vi "Ballistics Message Center.vi"(0 "INI File Name":string="ballistic.ini") -> ()   [LabVIEW 2015]
uses:
  Instance           1 33Saved   Ballistics Message Center .vi
panel:
  in  "Save":bool
  out "Over 10":string="Not Due"
  out "Over 9":string="Not Due"
  out "Over 8":string="Not Due"
  out "Over 7":string="Not Due"
  out "Over 6":string="Not Due"
  out "Over 5":string="Not Due"
  out "Over 4":string="Not Due"
  out "Over 3":string="Not Due"
  out "Over 2":string="Not Due"
  out "Over 1":string="Not Due"
  in  "Date":string[](array[string])
  in  "Interval in Days":string[](array[string])
  in  "Message":string[](array[string])
  in  "No Alarms":bool
  in  "Edit File":bool
  out "RadioArray":cluster{bool, bool}[](array[cluster])=[{FALSE, TRUE}, {FALSE, TRUE}, {FALSE, TRUE}, {FALSE, TRUE}, {FALSE, TRUE}, {FALSE, TRUE}, {FALSE, TRUE}, {FALSE, TRUE}, {FALSE, TRUE}, {FALSE, TRUE}]
  in  "Remind 1":bool=TRUE
  in  "Completed 1":bool
  out "Date 10":string
  out "Date 9":string
  out "Date 8":string
  out "Date 7":string
  out "Date 6":string
  out "Date 5":string
  out "Date 4":string
  out "Date 3":string
  out "Date 2":string
  out "Date 1":string
  in  "Remind 10":bool=TRUE
  in  "Remind 9":bool=TRUE
  in  "Remind 8":bool=TRUE
  in  "Remind 7":bool=TRUE
  in  "Remind 6":bool=TRUE
  in  "Remind 5":bool=TRUE
  in  "Remind 4":bool=TRUE
  in  "Remind 3":bool=TRUE
  in  "Remind 2":bool=TRUE
  in  "Completed 10":bool
  in  "Completed 9":bool
  in  "Completed 8":bool
  in  "Completed 7":bool
  in  "Completed 6":bool
  in  "Completed 5":bool
  in  "Completed 4":bool
  in  "Completed 3":bool
  in  "Completed 2":bool
  out "Message 10":string
  out "Message 9":string
  out "Message 8":string
  out "Message 7":string
  out "Message 6":string
  out "Message 5":string
  out "Message 4":string
  out "Message 3":string
  out "Message 2":string
  out "Message 1":string
  in  "Key Name":string[][](array[string])
  in  "Key Value":string[][](array[string])
  in  "Section Name":string="Reminders(10 max)"
  # "Days \nOverdue"
  # "Remind\nLater"
  # "Due Date"
  # "Complete"
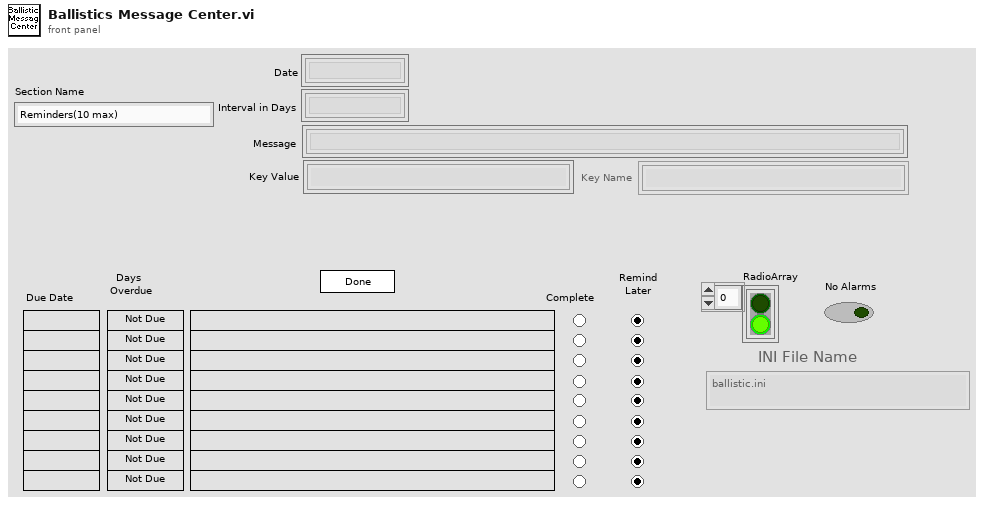
[diagram p1: front panel]
types:
  T1 = cluster{"second":i32, "minute":i32, "hour":i32, "day of month":i32, "month":i32, "year":i32, "day of week":i32, "day of year":i32, "is DST":i32}
  T2 = typedef "LVRectTypeDef.ctl" = cluster{"Left":i16, "Top":i16, "Right":i16, "Bottom":i16}
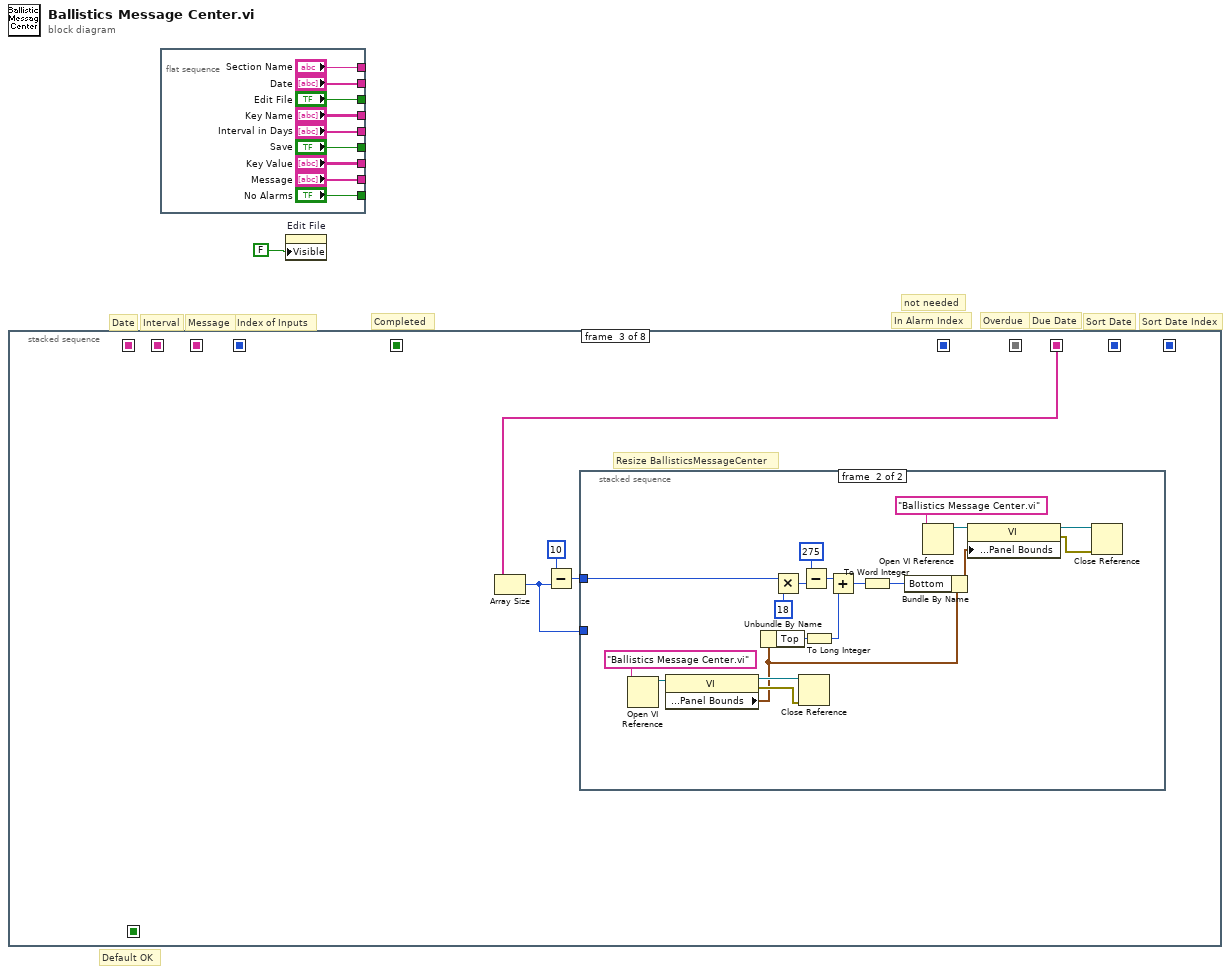
[diagram p0: block diagram]
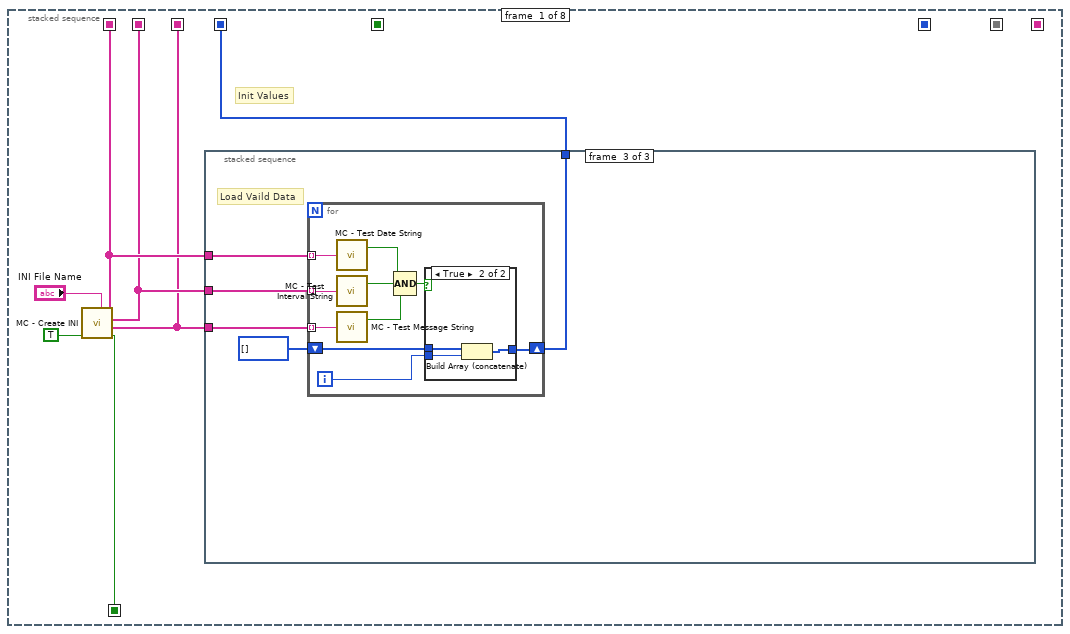
[diagram p2: hidden frame]
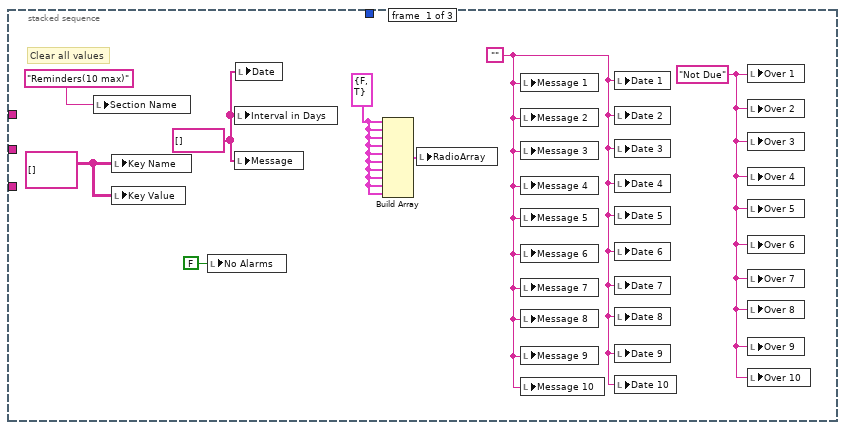
[diagram p3: hidden frame]
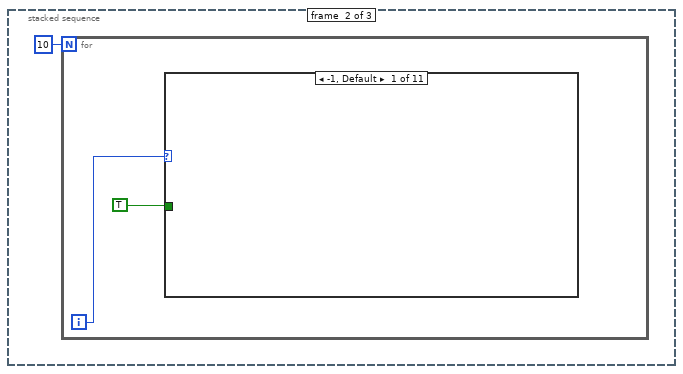
[diagram p4: hidden frame]
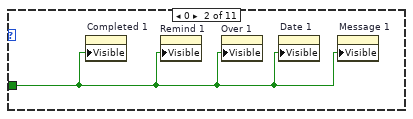
[diagram p5: hidden frame]
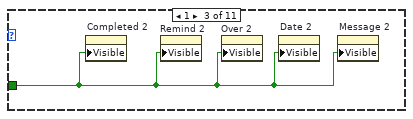
[diagram p6: hidden frame]
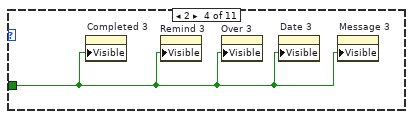
[diagram p7: hidden frame]
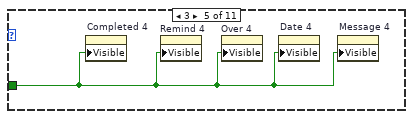
[diagram p8: hidden frame]
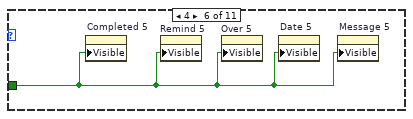
[diagram p9: hidden frame]
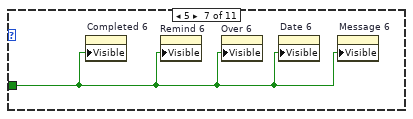
[diagram p10: hidden frame]
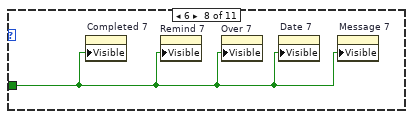
[diagram p11: hidden frame]
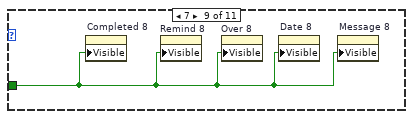
[diagram p12: hidden frame]
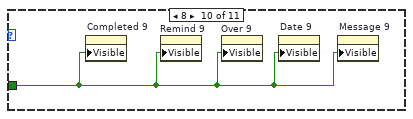
[diagram p13: hidden frame]
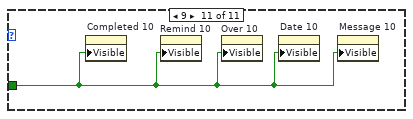
[diagram p14: hidden frame]
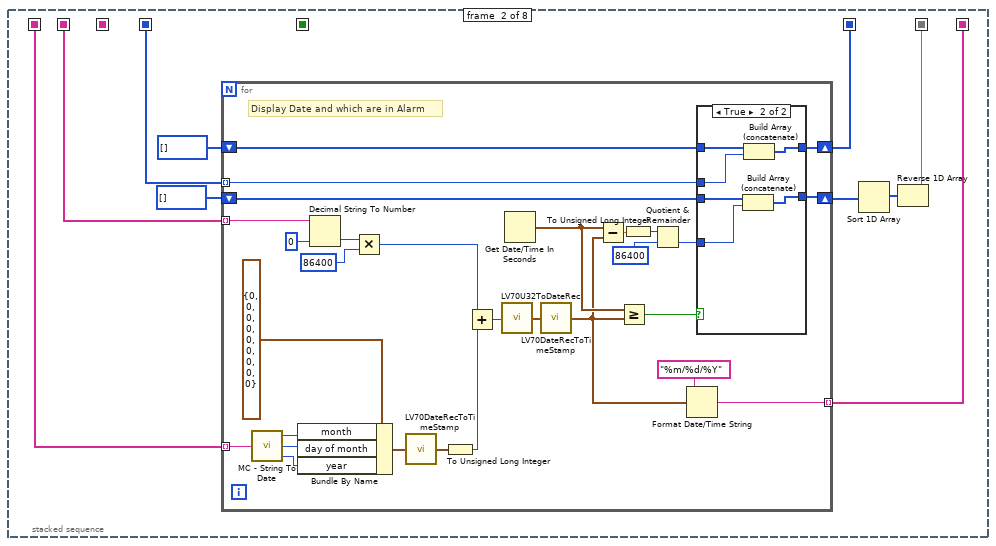
[diagram p16: hidden frame]
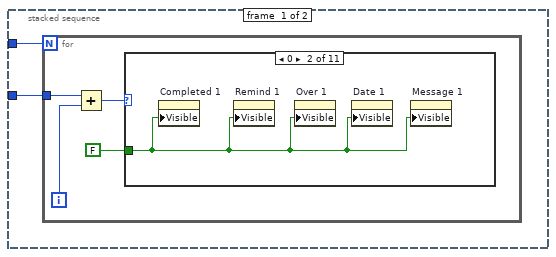
[diagram p18: hidden frame]
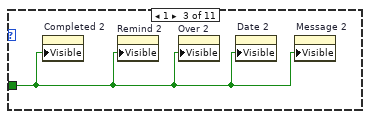
[diagram p20: hidden frame]
diagram:
  # "Default OK"
  # "not needed"
  # "Sort Date"
  # "Sort Date Index"
  # "Completed"
  # "Overdue"
  # "Index of Inputs"
  # "In Alarm Index"
  # "Due Date"
  # "Message"
  # "Interval"
  # "Date"
  n1 = stacked-sequence {
    seq-local: [_ _ _ _ _ _ w359 _] -> [_ _ _ _ _ _ _ w683]
    seq-local: [w6 _ _ _ _ _ _ _] -> [_ w57 _ _ _ _ _ w681]
    seq-local: [w5 _ _ _ _ _ _ _] -> [_ w58 _ _ _ _ _ w680]
    seq-local: [w4 _ _ _ _ _ _ _] -> [_ _ _ _ _ w212 _ w679]
    seq-local: [_ w54 _ _ _ _ _ _] -> [_ _ _ _ _ _ _ _]
    seq-local: [_ w53 _ _ _ _ _ _] -> [_ _ w99 w136 _ w211 _ _]
    seq-local: [w7 _ _ _ _ _ _ _] -> [_ w55 _ _ _ _ _ _]
    seq-local: [_ w49 _ _ _ _ _ _] -> [_ _ _ _ _ w210 _ _]
    seq-local: [_ _ _ w135 _ _ _ _] -> [_ _ _ _ w184 _ _ _]
    seq-local: [_ _ _ _ w185 _ _ _] -> [_ _ _ _ _ w209 _ w682]
    seq-local: [w3 _ _ _ _ _ _ _] -> [_ _ _ _ _ _ _ w678]
    frame #0 {
      # "Init Values"
      n2 = call "MC - Create INI.vi"("INI File Name"="INI File Name", "Save File"=TRUE) -> ("Default OK"=w3:bool, "Message Out"=w4:string[], "Interval in Days Out"=w5:string[], "Date Out"=w6:string[])  [unwired: 3 in, 1 out]
      n3 = stacked-sequence {
        tunnel: w6 -> [_ _ w33]
        tunnel: w5 -> [_ _ w32]
        tunnel: w4 -> [_ _ w31]
        tunnel: [_ _ w30] -> w7
        frame #0 {
          w10 = "Not Due"
          w11 = ""
          w12 = string[] [] ("Interval in Days")
          w15 = cluster{"Completed 10":bool, "Remind 10":bool} {"Completed 10"=FALSE, "Remind 10"=TRUE} ("input cluster")
          w16 = string[][] []
          # "Clear all values"
          n4 = local write "Section Name"("Reminders(10 max)") -> ()
          n5 = local write "Key Name"(w16) -> ()
          n6 = local write "Key Value"(w16) -> ()
          n7 = local write "No Alarms"(FALSE ("No Alarms")) -> ()
          n8 = local write "Interval in Days"(w12) -> ()
          n9 = local write "Message"(w12) -> ()
          n10 = local write "Date"(w12) -> ()
          n11 = Build Array(w15, w15, w15, w15, w15, w15, w15, w15, w15, w15) -> (w14:cluster{"Completed 10":bool, "Remind 10":bool}[])
          n12 = local write "RadioArray"(w14) -> ()
          n13 = local write "Message 1"(w11) -> ()
          n14 = local write "Message 2"(w11) -> ()
          n15 = local write "Message 3"(w11) -> ()
          n16 = local write "Message 4"(w11) -> ()
          n17 = local write "Message 5"(w11) -> ()
          n18 = local write "Message 6"(w11) -> ()
          n19 = local write "Message 7"(w11) -> ()
          n20 = local write "Message 8"(w11) -> ()
          n21 = local write "Message 9"(w11) -> ()
          n22 = local write "Message 10"(w11) -> ()
          n23 = local write "Date 1"(w11) -> ()
          n24 = local write "Date 2"(w11) -> ()
          n25 = local write "Date 3"(w11) -> ()
          n26 = local write "Date 4"(w11) -> ()
          n27 = local write "Date 5"(w11) -> ()
          n28 = local write "Date 6"(w11) -> ()
          n29 = local write "Date 7"(w11) -> ()
          n30 = local write "Date 8"(w11) -> ()
          n31 = local write "Date 9"(w11) -> ()
          n32 = local write "Date 10"(w11) -> ()
          n33 = local write "Over 1"(w10) -> ()
          n34 = local write "Over 2"(w10) -> ()
          n35 = local write "Over 3"(w10) -> ()
          n36 = local write "Over 4"(w10) -> ()
          n37 = local write "Over 5"(w10) -> ()
          n38 = local write "Over 6"(w10) -> ()
          n39 = local write "Over 7"(w10) -> ()
          n40 = local write "Over 8"(w10) -> ()
          n41 = local write "Over 9"(w10) -> ()
          n42 = local write "Over 10"(w10) -> ()
        }
        frame #1 {
          n43 = for {
            N: 10 -> [_]
            i -> [w18]
            n44 = case shown="-1, Default" w18 {
              tunnel: TRUE -> [_ w20 w21 w22 w23 w24 w25 w26 w27 w28 w29]
              frame -1, Default {
              }
              frame 0 {
                n45 = property on="Completed 1" class="Bool (strict)"("Visible"=w20) -> ()  [unwired: 2 in, 2 out]
                n46 = property on="Remind 1" class="Bool (strict)"("Visible"=w20) -> ()  [unwired: 2 in, 2 out]
                n47 = property on="Over 1" class="Str"("Visible"=w20) -> ()  [unwired: 2 in, 2 out]
                n48 = property on="Date 1" class="Str"("Visible"=w20) -> ()  [unwired: 2 in, 2 out]
                n49 = property on="Message 1" class="Str"("Visible"=w20) -> ()  [unwired: 2 in, 2 out]
              }
              frame 1 {
                n50 = property on="Completed 2" class="Bool (strict)"("Visible"=w21) -> ()  [unwired: 2 in, 2 out]
                n51 = property on="Remind 2" class="Bool (strict)"("Visible"=w21) -> ()  [unwired: 2 in, 2 out]
                n52 = property on="Over 2" class="Str"("Visible"=w21) -> ()  [unwired: 2 in, 2 out]
                n53 = property on="Date 2" class="Str"("Visible"=w21) -> ()  [unwired: 2 in, 2 out]
                n54 = property on="Message 2" class="Str"("Visible"=w21) -> ()  [unwired: 2 in, 2 out]
              }
              frame 2 {
                n55 = property on="Completed 3" class="Bool (strict)"("Visible"=w22) -> ()  [unwired: 2 in, 2 out]
                n56 = property on="Remind 3" class="Bool (strict)"("Visible"=w22) -> ()  [unwired: 2 in, 2 out]
                n57 = property on="Over 3" class="Str"("Visible"=w22) -> ()  [unwired: 2 in, 2 out]
                n58 = property on="Date 3" class="Str"("Visible"=w22) -> ()  [unwired: 2 in, 2 out]
                n59 = property on="Message 3" class="Str"("Visible"=w22) -> ()  [unwired: 2 in, 2 out]
              }
              frame 3 {
                n60 = property on="Completed 4" class="Bool (strict)"("Visible"=w23) -> ()  [unwired: 2 in, 2 out]
                n61 = property on="Remind 4" class="Bool (strict)"("Visible"=w23) -> ()  [unwired: 2 in, 2 out]
                n62 = property on="Over 4" class="Str"("Visible"=w23) -> ()  [unwired: 2 in, 2 out]
                n63 = property on="Date 4" class="Str"("Visible"=w23) -> ()  [unwired: 2 in, 2 out]
                n64 = property on="Message 4" class="Str"("Visible"=w23) -> ()  [unwired: 2 in, 2 out]
              }
              frame 4 {
                n65 = property on="Completed 5" class="Bool (strict)"("Visible"=w24) -> ()  [unwired: 2 in, 2 out]
                n66 = property on="Remind 5" class="Bool (strict)"("Visible"=w24) -> ()  [unwired: 2 in, 2 out]
                n67 = property on="Over 5" class="Str"("Visible"=w24) -> ()  [unwired: 2 in, 2 out]
                n68 = property on="Date 5" class="Str"("Visible"=w24) -> ()  [unwired: 2 in, 2 out]
                n69 = property on="Message 5" class="Str"("Visible"=w24) -> ()  [unwired: 2 in, 2 out]
              }
              frame 5 {
                n70 = property on="Completed 6" class="Bool (strict)"("Visible"=w25) -> ()  [unwired: 2 in, 2 out]
                n71 = property on="Remind 6" class="Bool (strict)"("Visible"=w25) -> ()  [unwired: 2 in, 2 out]
                n72 = property on="Over 6" class="Str"("Visible"=w25) -> ()  [unwired: 2 in, 2 out]
                n73 = property on="Date 6" class="Str"("Visible"=w25) -> ()  [unwired: 2 in, 2 out]
                n74 = property on="Message 6" class="Str"("Visible"=w25) -> ()  [unwired: 2 in, 2 out]
              }
              frame 6 {
                n75 = property on="Completed 7" class="Bool (strict)"("Visible"=w26) -> ()  [unwired: 2 in, 2 out]
                n76 = property on="Remind 7" class="Bool (strict)"("Visible"=w26) -> ()  [unwired: 2 in, 2 out]
                n77 = property on="Over 7" class="Str"("Visible"=w26) -> ()  [unwired: 2 in, 2 out]
                n78 = property on="Date 7" class="Str"("Visible"=w26) -> ()  [unwired: 2 in, 2 out]
                n79 = property on="Message 7" class="Str"("Visible"=w26) -> ()  [unwired: 2 in, 2 out]
              }
              frame 7 {
                n80 = property on="Completed 8" class="Bool (strict)"("Visible"=w27) -> ()  [unwired: 2 in, 2 out]
                n81 = property on="Remind 8" class="Bool (strict)"("Visible"=w27) -> ()  [unwired: 2 in, 2 out]
                n82 = property on="Over 8" class="Str"("Visible"=w27) -> ()  [unwired: 2 in, 2 out]
                n83 = property on="Date 8" class="Str"("Visible"=w27) -> ()  [unwired: 2 in, 2 out]
                n84 = property on="Message 8" class="Str"("Visible"=w27) -> ()  [unwired: 2 in, 2 out]
              }
              frame 8 {
                n85 = property on="Completed 9" class="Bool (strict)"("Visible"=w28) -> ()  [unwired: 2 in, 2 out]
                n86 = property on="Remind 9" class="Bool (strict)"("Visible"=w28) -> ()  [unwired: 2 in, 2 out]
                n87 = property on="Over 9" class="Str"("Visible"=w28) -> ()  [unwired: 2 in, 2 out]
                n88 = property on="Date 9" class="Str"("Visible"=w28) -> ()  [unwired: 2 in, 2 out]
                n89 = property on="Message 9" class="Str"("Visible"=w28) -> ()  [unwired: 2 in, 2 out]
              }
              frame 9 {
                n90 = property on="Completed 10" class="Bool (strict)"("Visible"=w29) -> ()  [unwired: 2 in, 2 out]
                n91 = property on="Remind 10" class="Bool (strict)"("Visible"=w29) -> ()  [unwired: 2 in, 2 out]
                n92 = property on="Over 10" class="Str"("Visible"=w29) -> ()  [unwired: 2 in, 2 out]
                n93 = property on="Date 10" class="Str"("Visible"=w29) -> ()  [unwired: 2 in, 2 out]
                n94 = property on="Message 10" class="Str"("Visible"=w29) -> ()  [unwired: 2 in, 2 out]
              }
            }
          }
        }
        frame #2 {
          # "Load Vaild Data"
          n95 = for {
            tunnel: w33 -> [w44] mode=indexing
            tunnel: w32 -> [w43] mode=indexing
            tunnel: w31 -> [w42] mode=indexing
            shift-right: [w35] -> w30
            shift-left: i32[] [] -> [w37]
            i -> [w36]
            n96 = call "MC - Test Date String.vi"("date string"=w44) -> ("valid date"=w41:bool)  [unwired: 1 out]
            n97 = call "MC - Test Interval String.vi"("interval string"=w43) -> ("valid interval"=w39:bool)  [unwired: 1 out]
            n98 = call "MC - Test Message String.vi"("message string"=w42) -> ("valid message"=w40:bool)  [unwired: 1 out]
            n99 = Compound Arithmetic op=AND(w41, w39, w40) -> (w38:bool)
            n100 = case shown="True" w38 {
              tunnel: w37 -> [w45 w48]
              tunnel: w36 -> [_ w47]
              tunnel: [w45 w46] -> w35
              frame False {
              }
              frame True {
                n101 = Build Array (concatenate)(w48, w47) -> (w46:i32[])
              }
            }
          }
        }
      }
    }
    frame #1 {
      n102 = for {
        tunnel: w58 -> [w74] mode=indexing
        tunnel: w57 -> [w73] mode=indexing
        tunnel: [w70] -> w53 mode=indexing
        shift-right: [w67] -> w54
        shift-left: i32[] [] -> [w69]
        tunnel: w55 -> [w68] mode=indexing
        shift-right: [w59] -> w51
        shift-left: u32[] [] -> [w61]
        # "Display Date and which are in Alarm"
        n103 = call "MC - String To Date.vi"("String Date"=w73) -> ("Month"=w86:u32, "Day"=w85:u32, "Year"=w84:u32)
        n104 = Bundle By Name(cluster=T1 {"second"=0, "minute"=0, "hour"=0, "day of month"=0, "month"=0, "year"=0, "day of week"=0, "day of year"=0, "is DST"=0} ("date time rec"), "month"=w86, "day of month"=w85, "year"=w84) -> (w83:T1)
        n105 = Decimal String To Number(string=w74, default (0L)=u32 0 ("Remind Check")) -> (number=w80:u32)  [unwired: 2 out]
        n106 = Multiply(x=w80, y=u32 86400 ("Remind Check")) -> (x*y=w71:u32)
        n107 = call <vilib>:"LV70DateRecToTimeStamp.vi"("date time rec"=w83) -> ("Time Stamp"=w77:timestamp)
        n108 = To Unsigned Long Integer(number=w77) -> (unsigned 32bit integer=w72:u32)
        n109 = Add(x=w71, y=w72) -> (x+y=w78:u32)
        n110 = call <vilib>:"LV70U32ToDateRec.vi"("Time"=w78) -> ("date time rec"=w76:T1)
        n111 = Get Date/Time In Seconds() -> (seconds since 1Jan1904=w66:timestamp)
        n112 = call <vilib>:"LV70DateRecToTimeStamp.vi"("date time rec"=w76) -> ("Time Stamp"=w65:timestamp)
        n113 = Subtract(x=w66, y=w65) -> (x-y=w64:dbl)
        n114 = Greater Or Equal?(x=w66, y=w65) -> (x >= y?=w82:bool)
        n115 = To Unsigned Long Integer(number=w64) -> (unsigned 32bit integer=w63:u32)
        n116 = Quotient & Remainder(x=w63, y=u32 86400 ("Remind Check")) -> (floor(x/y)=w60:u32)  [unwired: 1 out]
        n117 = Format Date/Time String(time format string (%c)="%m/%d/%Y", seconds (now)=w65) -> (date/time string=w70:string)  [unwired: 1 out]
        n118 = case shown="True" w82 {
          tunnel: w69 -> [w89 w95]
          tunnel: w68 -> [_ w94]
          tunnel: [w89 w93] -> w67
          tunnel: w61 -> [w88 w92]
          tunnel: w60 -> [_ w91]
          tunnel: [w88 w90] -> w59
          frame False {
          }
          frame True {
            n119 = Build Array (concatenate)(w92, w91) -> (w90:u32[])
            n120 = Build Array (concatenate)(w95, w94) -> (w93:i32[])
          }
        }
      }
      n121 = Sort 1D Array(array=w51) -> (sorted array=w50:u32[])
      n122 = Reverse 1D Array(array=w50) -> (reversed array=w49:u32[])
    }
    frame #2 {
      # "Resize BallisticsMessageCenter"
      n123 = Array Size(array=w99) -> (size(s)=w96:i32)
      n124 = Subtract(x=10, y=w96) -> (x-y=w97:i32)
      n125 = stacked-sequence {
        tunnel: w97 -> [w101 w132]
        tunnel: w96 -> [w100 _]
        frame #0 {
          n126 = for {
            N: w101 -> [_]
            tunnel: w100 -> [w105]
            i -> [w104]
            n127 = Add(x=w105, y=w104) -> (x+y=w103:i32)
            n128 = case shown="0" w103 {
              tunnel: FALSE -> [_ w106 w107 w108 w109 w110 w111 w112 w113 w114 w115]
              frame -1, Default {
              }
              frame 0 {
                n129 = property on="Completed 1" class="Bool (strict)"("Visible"=w106) -> ()  [unwired: 2 in, 2 out]
                n130 = property on="Remind 1" class="Bool (strict)"("Visible"=w106) -> ()  [unwired: 2 in, 2 out]
                n131 = property on="Over 1" class="Str"("Visible"=w106) -> ()  [unwired: 2 in, 2 out]
                n132 = property on="Date 1" class="Str"("Visible"=w106) -> ()  [unwired: 2 in, 2 out]
                n133 = property on="Message 1" class="Str"("Visible"=w106) -> ()  [unwired: 2 in, 2 out]
              }
              frame 1 {
                n134 = property on="Completed 2" class="Bool (strict)"("Visible"=w107) -> ()  [unwired: 2 in, 2 out]
                n135 = property on="Remind 2" class="Bool (strict)"("Visible"=w107) -> ()  [unwired: 2 in, 2 out]
                n136 = property on="Over 2" class="Str"("Visible"=w107) -> ()  [unwired: 2 in, 2 out]
                n137 = property on="Date 2" class="Str"("Visible"=w107) -> ()  [unwired: 2 in, 2 out]
                n138 = property on="Message 2" class="Str"("Visible"=w107) -> ()  [unwired: 2 in, 2 out]
              }
              frame 2 {
                n139 = property on="Completed 3" class="Bool (strict)"("Visible"=w108) -> ()  [unwired: 2 in, 2 out]
                n140 = property on="Remind 3" class="Bool (strict)"("Visible"=w108) -> ()  [unwired: 2 in, 2 out]
                n141 = property on="Over 3" class="Str"("Visible"=w108) -> ()  [unwired: 2 in, 2 out]
                n142 = property on="Date 3" class="Str"("Visible"=w108) -> ()  [unwired: 2 in, 2 out]
                n143 = property on="Message 3" class="Str"("Visible"=w108) -> ()  [unwired: 2 in, 2 out]
              }
              frame 3 {
                n144 = property on="Completed 4" class="Bool (strict)"("Visible"=w109) -> ()  [unwired: 2 in, 2 out]
                n145 = property on="Remind 4" class="Bool (strict)"("Visible"=w109) -> ()  [unwired: 2 in, 2 out]
                n146 = property on="Over 4" class="Str"("Visible"=w109) -> ()  [unwired: 2 in, 2 out]
                n147 = property on="Date 4" class="Str"("Visible"=w109) -> ()  [unwired: 2 in, 2 out]
                n148 = property on="Message 4" class="Str"("Visible"=w109) -> ()  [unwired: 2 in, 2 out]
              }
              frame 4 {
                n149 = property on="Completed 5" class="Bool (strict)"("Visible"=w110) -> ()  [unwired: 2 in, 2 out]
                n150 = property on="Remind 5" class="Bool (strict)"("Visible"=w110) -> ()  [unwired: 2 in, 2 out]
                n151 = property on="Over 5" class="Str"("Visible"=w110) -> ()  [unwired: 2 in, 2 out]
                n152 = property on="Date 5" class="Str"("Visible"=w110) -> ()  [unwired: 2 in, 2 out]
                n153 = property on="Message 5" class="Str"("Visible"=w110) -> ()  [unwired: 2 in, 2 out]
              }
              frame 5 {
                n154 = property on="Completed 6" class="Bool (strict)"("Visible"=w111) -> ()  [unwired: 2 in, 2 out]
                n155 = property on="Remind 6" class="Bool (strict)"("Visible"=w111) -> ()  [unwired: 2 in, 2 out]
                n156 = property on="Over 6" class="Str"("Visible"=w111) -> ()  [unwired: 2 in, 2 out]
                n157 = property on="Date 6" class="Str"("Visible"=w111) -> ()  [unwired: 2 in, 2 out]
                n158 = property on="Message 6" class="Str"("Visible"=w111) -> ()  [unwired: 2 in, 2 out]
              }
              frame 6 {
                n159 = property on="Completed 7" class="Bool (strict)"("Visible"=w112) -> ()  [unwired: 2 in, 2 out]
                n160 = property on="Remind 7" class="Bool (strict)"("Visible"=w112) -> ()  [unwired: 2 in, 2 out]
                n161 = property on="Over 7" class="Str"("Visible"=w112) -> ()  [unwired: 2 in, 2 out]
                n162 = property on="Date 7" class="Str"("Visible"=w112) -> ()  [unwired: 2 in, 2 out]
                n163 = property on="Message 7" class="Str"("Visible"=w112) -> ()  [unwired: 2 in, 2 out]
              }
              frame 7 {
                n164 = property on="Completed 8" class="Bool (strict)"("Visible"=w113) -> ()  [unwired: 2 in, 2 out]
                n165 = property on="Remind 8" class="Bool (strict)"("Visible"=w113) -> ()  [unwired: 2 in, 2 out]
                n166 = property on="Over 8" class="Str"("Visible"=w113) -> ()  [unwired: 2 in, 2 out]
                n167 = property on="Date 8" class="Str"("Visible"=w113) -> ()  [unwired: 2 in, 2 out]
                n168 = property on="Message 8" class="Str"("Visible"=w113) -> ()  [unwired: 2 in, 2 out]
              }
              frame 8 {
                n169 = property on="Completed 9" class="Bool (strict)"("Visible"=w114) -> ()  [unwired: 2 in, 2 out]
                n170 = property on="Remind 9" class="Bool (strict)"("Visible"=w114) -> ()  [unwired: 2 in, 2 out]
                n171 = property on="Over 9" class="Str"("Visible"=w114) -> ()  [unwired: 2 in, 2 out]
                n172 = property on="Date 9" class="Str"("Visible"=w114) -> ()  [unwired: 2 in, 2 out]
                n173 = property on="Message 9" class="Str"("Visible"=w114) -> ()  [unwired: 2 in, 2 out]
              }
              frame 9 {
                n174 = property on="Completed 10" class="Bool (strict)"("Visible"=w115) -> ()  [unwired: 2 in, 2 out]
                n175 = property on="Remind 10" class="Bool (strict)"("Visible"=w115) -> ()  [unwired: 2 in, 2 out]
                n176 = property on="Over 10" class="Str"("Visible"=w115) -> ()  [unwired: 2 in, 2 out]
                n177 = property on="Date 10" class="Str"("Visible"=w115) -> ()  [unwired: 2 in, 2 out]
                n178 = property on="Message 10" class="Str"("Visible"=w115) -> ()  [unwired: 2 in, 2 out]
              }
            }
          }
        }
        frame #1 {
          n179 = Open VI Reference(vi path="Ballistics Message Center.vi") -> (vi reference=w133:refnum<vi>)  [unwired: 1 in, 5 out]
          n180 = property class="VI"(reference=w133) -> (reference out=w126:refnum<vi>, error out=w125:errorcluster, "Front Panel Window:Panel Bounds"=w116:T2)  [unwired: 1 in]
          n181 = Unbundle By Name(w116) -> ("Top"=w127:i16)
          n182 = Multiply(x=w132, y=18) -> (x*y=w130:i32)
          n183 = Close Reference(reference=w126, error in (no error)=w125) -> ()  [unwired: 1 out]
          n184 = Subtract(x=275, y=w130) -> (x-y=w128:i32)
          n185 = To Long Integer(number=w127) -> (32bit integer=w124:i32)
          n186 = Add(x=w128, y=w124) -> (x+y=w117:i32)
          n187 = To Word Integer(number=w117) -> (16bit integer=w118:i16)
          n188 = Bundle By Name(cluster=w116, "Bottom"=w118) -> (w121:T2)
          n189 = Open VI Reference(vi path="Ballistics Message Center.vi") -> (vi reference=w122:refnum<vi>)  [unwired: 1 in, 5 out]
          n190 = property class="VI"(reference=w122, "Front Panel Window:Panel Bounds"=w121) -> (reference out=w120:refnum<vi>, error out=w119:errorcluster)  [unwired: 1 in]
          n191 = Close Reference(reference=w120, error in (no error)=w119) -> ()  [unwired: 1 out]
        }
      }
    }
    frame #3 {
      n192 = Array Size(array=w136) -> (size(s)=w137:i32)
      n193 = for {
        N: w137 -> [_]
        tunnel: w136 -> [w140]
        tunnel: [w138] -> w135 mode=indexing
        i -> [w142]
        n194 = Index Array(array=w140, index=w142) -> (element=w146:string)
        n195 = call "MC - String To Date.vi"("String Date"=w146) -> ("Month"=w151:u32, "Day"=w150:u32, "Year"=w149:u32)
        n196 = Bundle By Name(cluster=T1 {"second"=0, "minute"=0, "hour"=0, "day of month"=0, "month"=0, "year"=0, "day of week"=0, "day of year"=0, "is DST"=0} ("date time rec"), "month"=w151, "day of month"=w150, "year"=w149) -> (w148:T1)
        n197 = Array Size(array=w140) -> (size(s)=w145:i32)
        n198 = call <vilib>:"LV70DateRecToTimeStamp.vi"("date time rec"=w148) -> ("Time Stamp"=w147:timestamp)
        n199 = Decrement(x=w145) -> (x-1=w144:i32)
        n200 = To Unsigned Long Integer(number=w147) -> (unsigned 32bit integer=w141:u32)
        n201 = for {
          N: w144 -> [_]
          tunnel: w140 -> [w171]
          shift-right: [w166] -> _
          shift-left: 0 -> [w170]
          tunnel: w142 -> [w168]
          tunnel: w141 -> [w156]
          shift-right: [w153] -> w138
          shift-left: 0 -> [w154]
          i -> [w167]
          n202 = Equal?(x=w167, y=w168) -> (x = y?=w169:bool)
          n203 = case shown="True" w169 {
            tunnel: w170 -> [w175 w177]
            tunnel: [w175 w176] -> w166
            frame False {
            }
            frame True {
              n204 = Increment(x=w177) -> (x+1=w176:i32)
            }
          }
          n205 = Add(x=w167, y=w166) -> (x+y=w165:i32)
          n206 = Index Array(array=w171, index=w165) -> (element=w158:string)
          n207 = call "MC - String To Date.vi"("String Date"=w158) -> ("Month"=w160:u32, "Day"=w161:u32, "Year"=w162:u32)
          n208 = Bundle By Name(cluster=T1 {"second"=0, "minute"=0, "hour"=0, "day of month"=0, "month"=0, "year"=0, "day of week"=0, "day of year"=0, "is DST"=0} ("date time rec"), "month"=w160, "day of month"=w161, "year"=w162) -> (w163:T1)
          n209 = call <vilib>:"LV70DateRecToTimeStamp.vi"("date time rec"=w163) -> ("Time Stamp"=w164:timestamp)
          n210 = To Unsigned Long Integer(number=w164) -> (unsigned 32bit integer=w157:u32)
          n211 = Greater Or Equal?(x=w156, y=w157) -> (x >= y?=w155:bool)
          n212 = case shown="True" w155 {
            tunnel: w154 -> [w172 w174]
            tunnel: [w172 w173] -> w153
            frame False {
            }
            frame True {
              n213 = Increment(x=w174) -> (x+1=w173:i32)
            }
          }
        }
      }
    }
    frame #4 {
      # "Link sorted date to original index"
      n214 = Array Size(array=w184) -> (size(s)=w181:i32)
      n215 = Array Size(array=w184) -> (size(s)=w182:i32)
      n216 = Multiply(x=w182, y=w181) -> (x*y=w183:i32)
      n217 = for {
        N: w183 -> [_]
        tunnel: w184 -> [w196]
        tunnel: w181 -> [w197]
        shift-right: [w192] -> _
        shift-left: 0 -> [w194]
        shift-right: [w189] -> _
        shift-left: 0 -> [w188]
        shift-right: [w186] -> w185
        shift-left: i32[] [] -> [w187]
        i -> [w198]
        n218 = Quotient & Remainder(x=w198, y=w197) -> (floor(x/y)=w190:i32)  [unwired: 1 out]
        n219 = Equal?(x=w190, y=w188) -> (x = y?=w195:bool)
        n220 = case shown="True" w195 {
          tunnel: w194 -> [_ w202]
          tunnel: [0 w202] -> w193
          tunnel: w190 -> [w199 _]
          tunnel: [w199 w201] -> w189
          tunnel: w188 -> [_ w201]
          frame False {
          }
          frame True {
          }
        }
        n221 = Search 1D Array(1D array=w196, element=w190, start index (0)=w193) -> (index of element=w191:i32)
        n222 = case shown="0.." w191 {
          tunnel: w193 -> [w204 _]
          tunnel: [w204 w208] -> w192
          tunnel: w191 -> [_ w206]
          tunnel: w187 -> [w203 w207]
          tunnel: [w203 w205] -> w186
          frame ..-1 {
          }
          frame 0.. {
            n223 = Build Array (concatenate)(w207, w206) -> (w205:i32[])
            n224 = Increment(x=w206) -> (x+1=w208:i32)
          }
        }
      }
    }
    frame #5 {
      # "Sorted Message"
      # "Sorted Due Date"
      # "Fill front panel"
      n225 = stacked-sequence {
        seq-local: [w214 _ _] -> [_ _ w324]
        tunnel: w210 -> [w213 _ _]
        tunnel: w212 -> [_ w294 _]
        tunnel: w211 -> [_ w295 _]
        tunnel: w209 -> [_ w291 _]
        frame #0 {
          n226 = local read "RadioArray"() -> (w215:cluster{bool, bool}[])
          n227 = for {
            tunnel: w213 -> [w216] mode=indexing
            shift-right: [w218] -> w214
            shift-left: w215 -> [w219]
            i -> [w217]
            # "Set Alarm Buttons"
            n228 = case shown="9" w217 {
              selector: w217 -> [_ w227 w234 w241 w248 w255 w262 w269 w276 w283 w290]
              tunnel: w219 -> [w220 w225 w232 w239 w246 w253 w260 w267 w274 w281 w288]
              tunnel: [w220 w224 w231 w238 w245 w252 w259 w266 w273 w280 w287] -> w218
              tunnel: w216 -> [_ w221 w229 w236 w243 w250 w257 w264 w271 w278 w285]
              frame -1, Default {
              }
              frame 0 {
                n229 = Format Into String(w221) -> (resulting string=→"Over 1":string)  [unwired: 3 in, 1 out]
                n230 = Insert Into Array(array=w225, index=w227, new element=cluster{"Completed 10":bool, "Remind 10":bool} {"Completed 10"=FALSE, "Remind 10"=FALSE} ("input cluster")) -> (w224:cluster{bool, bool}[])
                n231 = property on="Date 1" class="Str"("Blinking"=TRUE) -> ()  [unwired: 2 in, 2 out]
              }
              frame 1 {
                n232 = Format Into String(w229) -> (resulting string=→"Over 2":string)  [unwired: 3 in, 1 out]
                n233 = Insert Into Array(array=w232, index=w234, new element=cluster{"Completed 10":bool, "Remind 10":bool} {"Completed 10"=FALSE, "Remind 10"=FALSE} ("input cluster")) -> (w231:cluster{bool, bool}[])
                n234 = property on="Date 2" class="Str"("Blinking"=TRUE) -> ()  [unwired: 2 in, 2 out]
              }
              frame 2 {
                n235 = Format Into String(w236) -> (resulting string=→"Over 3":string)  [unwired: 3 in, 1 out]
                n236 = Insert Into Array(array=w239, index=w241, new element=cluster{"Completed 10":bool, "Remind 10":bool} {"Completed 10"=FALSE, "Remind 10"=FALSE} ("input cluster")) -> (w238:cluster{bool, bool}[])
                n237 = property on="Date 3" class="Str"("Blinking"=TRUE) -> ()  [unwired: 2 in, 2 out]
              }
              frame 3 {
                n238 = Format Into String(w243) -> (resulting string=→"Over 4":string)  [unwired: 3 in, 1 out]
                n239 = Insert Into Array(array=w246, index=w248, new element=cluster{"Completed 10":bool, "Remind 10":bool} {"Completed 10"=FALSE, "Remind 10"=FALSE} ("input cluster")) -> (w245:cluster{bool, bool}[])
                n240 = property on="Date 4" class="Str"("Blinking"=TRUE) -> ()  [unwired: 2 in, 2 out]
              }
              frame 4 {
                n241 = Format Into String(w250) -> (resulting string=→"Over 5":string)  [unwired: 3 in, 1 out]
                n242 = Insert Into Array(array=w253, index=w255, new element=cluster{"Completed 10":bool, "Remind 10":bool} {"Completed 10"=FALSE, "Remind 10"=FALSE} ("input cluster")) -> (w252:cluster{bool, bool}[])
                n243 = property on="Date 5" class="Str"("Blinking"=TRUE) -> ()  [unwired: 2 in, 2 out]
              }
              frame 5 {
                n244 = Format Into String(w257) -> (resulting string=→"Over 6":string)  [unwired: 3 in, 1 out]
                n245 = Insert Into Array(array=w260, index=w262, new element=cluster{"Completed 10":bool, "Remind 10":bool} {"Completed 10"=FALSE, "Remind 10"=FALSE} ("input cluster")) -> (w259:cluster{bool, bool}[])
                n246 = property on="Date 6" class="Str"("Blinking"=TRUE) -> ()  [unwired: 2 in, 2 out]
              }
              frame 6 {
                n247 = Format Into String(w264) -> (resulting string=→"Over 7":string)  [unwired: 3 in, 1 out]
                n248 = Insert Into Array(array=w267, index=w269, new element=cluster{"Completed 10":bool, "Remind 10":bool} {"Completed 10"=FALSE, "Remind 10"=FALSE} ("input cluster")) -> (w266:cluster{bool, bool}[])
                n249 = property on="Date 7" class="Str"("Blinking"=TRUE) -> ()  [unwired: 2 in, 2 out]
              }
              frame 7 {
                n250 = Format Into String(w271) -> (resulting string=→"Over 8":string)  [unwired: 3 in, 1 out]
                n251 = Insert Into Array(array=w274, index=w276, new element=cluster{"Completed 10":bool, "Remind 10":bool} {"Completed 10"=FALSE, "Remind 10"=FALSE} ("input cluster")) -> (w273:cluster{bool, bool}[])
                n252 = property on="Date 8" class="Str"("Blinking"=TRUE) -> ()  [unwired: 2 in, 2 out]
              }
              frame 8 {
                n253 = Format Into String(w278) -> (resulting string=→"Over 9":string)  [unwired: 3 in, 1 out]
                n254 = Insert Into Array(array=w281, index=w283, new element=cluster{"Completed 10":bool, "Remind 10":bool} {"Completed 10"=FALSE, "Remind 10"=FALSE} ("input cluster")) -> (w280:cluster{bool, bool}[])
                n255 = property on="Date 9" class="Str"("Blinking"=TRUE) -> ()  [unwired: 2 in, 2 out]
              }
              frame 9 {
                n256 = Format Into String(w285) -> (resulting string=→"Over 10":string)  [unwired: 3 in, 1 out]
                n257 = Insert Into Array(array=w288, index=w290, new element=cluster{"Completed 10":bool, "Remind 10":bool} {"Completed 10"=FALSE, "Remind 10"=FALSE} ("input cluster")) -> (w287:cluster{bool, bool}[])
                n258 = property on="Date 10" class="Str"("Blinking"=TRUE) -> ()  [unwired: 2 in, 2 out]
              }
            }
          }
          "RadioArray" <- w214
        }
        frame #1 {
          # "Message"
          # "Date"
          n259 = for {
            tunnel: w291 -> [w321] mode=indexing
            tunnel: w295 -> [w323]
            tunnel: w294 -> [w322]
            tunnel: [w320] -> w292 mode=indexing
            tunnel: [w319] -> w293 mode=indexing
            n260 = Index Array(array=w322, index=w321) -> (element=w320:string)
            n261 = Index Array(array=w323, index=w321) -> (element=w319:string)
          }
          n262 = for {
            tunnel: w293 -> [w297] mode=indexing
            tunnel: w292 -> [w296] mode=indexing
            i -> [w298]
            n263 = case shown="9" w298 {
              tunnel: w297 -> [_ w300 w302 w304 w306 w308 w310 w312 w314 w316 w318]
              tunnel: w296 -> [_ w299 w301 w303 w305 w307 w309 w311 w313 w315 w317]
              frame -1, Default {
              }
              frame 0 {
                "Date 1" <- w300
                "Message 1" <- w299
              }
              frame 1 {
                "Date 2" <- w302
                "Message 2" <- w301
              }
              frame 2 {
                "Date 3" <- w304
                "Message 3" <- w303
              }
              frame 3 {
                "Date 4" <- w306
                "Message 4" <- w305
              }
              frame 4 {
                "Date 5" <- w308
                "Message 5" <- w307
              }
              frame 5 {
                "Date 6" <- w310
                "Message 6" <- w309
              }
              frame 6 {
                "Date 7" <- w312
                "Message 7" <- w311
              }
              frame 7 {
                "Date 8" <- w314
                "Message 8" <- w313
              }
              frame 8 {
                "Date 9" <- w316
                "Message 9" <- w315
              }
              frame 9 {
                "Date 10" <- w318
                "Message 10" <- w317
              }
            }
          }
        }
        frame #2 {
          n264 = for {
            tunnel: w324 -> [w325] mode=indexing
            i -> [w326]
            n265 = case shown="0" w326 {
              tunnel: w325 -> [_ w329 w332 w335 w338 w341 w344 w347 w350 w353 w356]
              frame -1, Default {
              }
              frame 0 {
                n266 = Unbundle(w329) -> (w328:bool, w327:bool)
                n267 = local write "Completed 1"(w328) -> ()
                n268 = local write "Remind 1"(w327) -> ()
              }
              frame 1 {
                n269 = Unbundle(w332) -> (w331:bool, w330:bool)
                n270 = local write "Completed 2"(w331) -> ()
                n271 = local write "Remind 2"(w330) -> ()
              }
              frame 2 {
                n272 = Unbundle(w335) -> (w334:bool, w333:bool)
                n273 = local write "Completed 3"(w334) -> ()
                n274 = local write "Remind 3"(w333) -> ()
              }
              frame 3 {
                n275 = Unbundle(w338) -> (w337:bool, w336:bool)
                n276 = local write "Completed 4"(w337) -> ()
                n277 = local write "Remind 4"(w336) -> ()
              }
              frame 4 {
                n278 = Unbundle(w341) -> (w340:bool, w339:bool)
                n279 = local write "Completed 5"(w340) -> ()
                n280 = local write "Remind 5"(w339) -> ()
              }
              frame 5 {
                n281 = Unbundle(w344) -> (w343:bool, w342:bool)
                n282 = local write "Completed 6"(w343) -> ()
                n283 = local write "Remind 6"(w342) -> ()
              }
              frame 6 {
                n284 = Unbundle(w347) -> (w346:bool, w345:bool)
                n285 = local write "Completed 7"(w346) -> ()
                n286 = local write "Remind 7"(w345) -> ()
              }
              frame 7 {
                n287 = Unbundle(w350) -> (w349:bool, w348:bool)
                n288 = local write "Completed 8"(w349) -> ()
                n289 = local write "Remind 8"(w348) -> ()
              }
              frame 8 {
                n290 = Unbundle(w353) -> (w352:bool, w351:bool)
                n291 = local write "Completed 9"(w352) -> ()
                n292 = local write "Remind 9"(w351) -> ()
              }
              frame 9 {
                n293 = Unbundle(w356) -> (w355:bool, w354:bool)
                n294 = local write "Completed 10"(w355) -> ()
                n295 = local write "Remind 10"(w354) -> ()
              }
            }
          }
        }
      }
    }
    frame #6 {
      n296 = local read "RadioArray"() -> (w360:cluster{bool, bool}[])
      n297 = property on="Save" class="Bool (strict)"("Visible"=TRUE) -> (error out=w357:errorcluster)  [unwired: 2 in, 1 out]
      n298 = while {
        shift-right: [w364] -> _
        shift-left: w360 -> [w363]
        tunnel: [w361] -> w359
        tunnel: w357 -> [_]
        stop <- w362 stop-if-true
        # "Com or Rem"
        # "Remind"
        n299 = stacked-sequence {
          seq-local: [w367 _ _ _ _] -> [_ w600 _ _ _]
          seq-local: [_ w598 _ _ _] -> [_ _ w659 _ _]
          seq-local: [_ w597 _ _ _] -> [_ _ _ _ w670]
          tunnel: [w367 _ _ _ _] -> w364
          tunnel: w363 -> [w366 _ _ _ _]
          tunnel: [_ _ _ _ w666] -> w362
          tunnel: [_ w599 _ _ _] -> w361
          frame #0 {
            n300 = stacked-sequence {
              tunnel: [_ _ _ _ _ _ _ _ _ _ _ _ _ _ _ _ _ _ _ _ _ w563 _ _ _ _ _ _ _ _] -> w376
              tunnel: [_ _ _ _ _ _ _ _ _ _ _ _ _ _ _ _ _ _ _ _ _ _ w565 _ _ _ _ _ _ _] -> w375
              tunnel: [_ _ _ _ _ _ _ _ _ _ _ _ _ _ _ _ _ _ _ _ _ _ _ w569 _ _ _ _ _ _] -> w374
              tunnel: [_ _ _ _ _ _ _ _ _ _ _ _ _ _ _ _ _ _ _ _ _ _ _ _ w573 _ _ _ _ _] -> w373
              tunnel: [_ _ _ _ _ _ _ _ _ _ _ _ _ _ _ _ _ _ _ _ _ _ _ _ _ w577 _ _ _ _] -> w372
              tunnel: [_ _ _ _ _ _ _ _ _ _ _ _ _ _ _ _ _ _ _ _ _ _ _ _ _ _ w581 _ _ _] -> w371
              tunnel: [_ _ _ _ _ _ _ _ _ _ _ _ _ _ _ _ _ _ _ _ _ _ _ _ _ _ _ w585 _ _] -> w370
              tunnel: [_ _ _ _ _ _ _ _ _ _ _ _ _ _ _ _ _ _ _ _ _ _ _ _ _ _ _ _ w589 _] -> w369
              tunnel: [_ _ _ _ _ _ _ _ _ _ _ _ _ _ _ _ _ _ _ _ _ _ _ _ _ _ _ _ _ w593] -> w368
              tunnel: w366 -> [w380 w389 w398 w407 w416 w425 w434 w443 w452 w461 w470 w479 w488 w497 w506 w515 w524 w533 w542 w551 _ _ _ _ _ _ _ _ _ _]
              tunnel: [_ _ _ _ _ _ _ _ _ _ _ _ _ _ _ _ _ _ _ _ w557 _ _ _ _ _ _ _ _ _] -> w365
              frame #0 {
                # "Make like Option Buttons"
                n301 = Index Array(array=w380, index=0) -> (element=w378:cluster{bool, bool})
                n302 = Unbundle(w378) -> (w377:bool)  [unwired: 1 out]
                n303 = stacked-sequence {
                  tunnel: w377 -> [w381]
                  frame #0 {
                    n304 = case shown="False" w381 {
                      frame False {
                        n305 = local read "Completed 1"() -> (w382:bool)
                        n306 = case shown="True" w382 {
                          frame False {
                            n307 = property on="Completed 1" class="Bool (strict)"("Disabled"=u8 0) -> ()  [unwired: 2 in, 2 out]
                          }
                          frame True {
                            n308 = local write "Remind 1"(FALSE ("y")) -> ()
                            n309 = property on="Completed 1" class="Bool (strict)"("Disabled"=u8 1) -> ()  [unwired: 2 in, 2 out]
                          }
                        }
                      }
                      frame True {
                      }
                    }
                  }
                }
              }
              frame #1 {
                n310 = Index Array(array=w389, index=1) -> (element=w387:cluster{bool, bool})
                n311 = Unbundle(w387) -> (w386:bool)  [unwired: 1 out]
                n312 = stacked-sequence {
                  tunnel: w386 -> [w390]
                  frame #0 {
                    n313 = case shown="False" w390 {
                      frame False {
                        n314 = local read "Completed 2"() -> (w391:bool)
                        n315 = case shown="True" w391 {
                          frame False {
                            n316 = property on="Completed 2" class="Bool (strict)"("Disabled"=u8 0) -> ()  [unwired: 2 in, 2 out]
                          }
                          frame True {
                            n317 = local write "Remind 2"(FALSE ("y")) -> ()
                            n318 = property on="Completed 2" class="Bool (strict)"("Disabled"=u8 1) -> ()  [unwired: 2 in, 2 out]
                          }
                        }
                      }
                      frame True {
                      }
                    }
                  }
                }
              }
              frame #2 {
                n319 = Index Array(array=w398, index=2) -> (element=w396:cluster{bool, bool})
                n320 = Unbundle(w396) -> (w395:bool)  [unwired: 1 out]
                n321 = stacked-sequence {
                  tunnel: w395 -> [w399]
                  frame #0 {
                    n322 = case shown="False" w399 {
                      frame False {
                        n323 = local read "Completed 3"() -> (w400:bool)
                        n324 = case shown="True" w400 {
                          frame False {
                            n325 = property on="Completed 3" class="Bool (strict)"("Disabled"=u8 0) -> ()  [unwired: 2 in, 2 out]
                          }
                          frame True {
                            n326 = local write "Remind 3"(FALSE ("y")) -> ()
                            n327 = property on="Completed 3" class="Bool (strict)"("Disabled"=u8 1) -> ()  [unwired: 2 in, 2 out]
                          }
                        }
                      }
                      frame True {
                      }
                    }
                  }
                }
              }
              frame #3 {
                n328 = Index Array(array=w407, index=3) -> (element=w405:cluster{bool, bool})
                n329 = Unbundle(w405) -> (w404:bool)  [unwired: 1 out]
                n330 = stacked-sequence {
                  tunnel: w404 -> [w408]
                  frame #0 {
                    n331 = case shown="False" w408 {
                      frame False {
                        n332 = local read "Completed 4"() -> (w409:bool)
                        n333 = case shown="False" w409 {
                          frame False {
                            n334 = property on="Completed 4" class="Bool (strict)"("Disabled"=u8 0) -> ()  [unwired: 2 in, 2 out]
                          }
                          frame True {
                            n335 = local write "Remind 4"(FALSE ("y")) -> ()
                            n336 = property on="Completed 4" class="Bool (strict)"("Disabled"=u8 1) -> ()  [unwired: 2 in, 2 out]
                          }
                        }
                      }
                      frame True {
                      }
                    }
                  }
                }
              }
              frame #4 {
                n337 = Index Array(array=w416, index=4) -> (element=w414:cluster{bool, bool})
                n338 = Unbundle(w414) -> (w413:bool)  [unwired: 1 out]
                n339 = stacked-sequence {
                  tunnel: w413 -> [w417]
                  frame #0 {
                    n340 = case shown="False" w417 {
                      frame False {
                        n341 = local read "Completed 5"() -> (w418:bool)
                        n342 = case shown="True" w418 {
                          frame False {
                            n343 = property on="Completed 5" class="Bool (strict)"("Disabled"=u8 0) -> ()  [unwired: 2 in, 2 out]
                          }
                          frame True {
                            n344 = local write "Remind 5"(FALSE ("y")) -> ()
                            n345 = property on="Completed 5" class="Bool (strict)"("Disabled"=u8 1) -> ()  [unwired: 2 in, 2 out]
                          }
                        }
                      }
                      frame True {
                      }
                    }
                  }
                }
              }
              frame #5 {
                n346 = Index Array(array=w425, index=5) -> (element=w423:cluster{bool, bool})
                n347 = Unbundle(w423) -> (w422:bool)  [unwired: 1 out]
                n348 = stacked-sequence {
                  tunnel: w422 -> [w426]
                  frame #0 {
                    n349 = case shown="False" w426 {
                      frame False {
                        n350 = local read "Completed 6"() -> (w427:bool)
                        n351 = case shown="True" w427 {
                          frame False {
                            n352 = property on="Completed 6" class="Bool (strict)"("Disabled"=u8 0) -> ()  [unwired: 2 in, 2 out]
                          }
                          frame True {
                            n353 = local write "Remind 6"(FALSE ("y")) -> ()
                            n354 = property on="Completed 6" class="Bool (strict)"("Disabled"=u8 1) -> ()  [unwired: 2 in, 2 out]
                          }
                        }
                      }
                      frame True {
                      }
                    }
                  }
                }
              }
              frame #6 {
                n355 = Index Array(array=w434, index=6) -> (element=w432:cluster{bool, bool})
                n356 = Unbundle(w432) -> (w431:bool)  [unwired: 1 out]
                n357 = stacked-sequence {
                  tunnel: w431 -> [w435]
                  frame #0 {
                    n358 = case shown="False" w435 {
                      frame False {
                        n359 = local read "Completed 7"() -> (w436:bool)
                        n360 = case shown="False" w436 {
                          frame False {
                            n361 = property on="Completed 7" class="Bool (strict)"("Disabled"=u8 0) -> ()  [unwired: 2 in, 2 out]
                          }
                          frame True {
                            n362 = property on="Completed 7" class="Bool (strict)"("Disabled"=u8 1) -> ()  [unwired: 2 in, 2 out]
                            n363 = local write "Remind 7"(FALSE ("y")) -> ()
                          }
                        }
                      }
                      frame True {
                      }
                    }
                  }
                }
              }
              frame #7 {
                n364 = Index Array(array=w443, index=7) -> (element=w441:cluster{bool, bool})
                n365 = Unbundle(w441) -> (w440:bool)  [unwired: 1 out]
                n366 = stacked-sequence {
                  tunnel: w440 -> [w444]
                  frame #0 {
                    n367 = case shown="False" w444 {
                      frame False {
                        n368 = local read "Completed 8"() -> (w445:bool)
                        n369 = case shown="True" w445 {
                          frame False {
                            n370 = property on="Completed 8" class="Bool (strict)"("Disabled"=u8 0) -> ()  [unwired: 2 in, 2 out]
                          }
                          frame True {
                            n371 = local write "Remind 8"(FALSE ("y")) -> ()
                            n372 = property on="Completed 8" class="Bool (strict)"("Disabled"=u8 1) -> ()  [unwired: 2 in, 2 out]
                          }
                        }
                      }
                      frame True {
                      }
                    }
                  }
                }
              }
              frame #8 {
                n373 = Index Array(array=w452, index=8) -> (element=w450:cluster{bool, bool})
                n374 = Unbundle(w450) -> (w449:bool)  [unwired: 1 out]
                n375 = stacked-sequence {
                  tunnel: w449 -> [w453]
                  frame #0 {
                    n376 = case shown="False" w453 {
                      frame False {
                        n377 = local read "Completed 9"() -> (w454:bool)
                        n378 = case shown="False" w454 {
                          frame False {
                            n379 = property on="Completed 9" class="Bool (strict)"("Disabled"=u8 0) -> ()  [unwired: 2 in, 2 out]
                          }
                          frame True {
                            n380 = local write "Remind 9"(FALSE ("y")) -> ()
                            n381 = property on="Completed 9" class="Bool (strict)"("Disabled"=u8 1) -> ()  [unwired: 2 in, 2 out]
                          }
                        }
                      }
                      frame True {
                      }
                    }
                  }
                }
              }
              frame #9 {
                n382 = Index Array(array=w461, index=9) -> (element=w459:cluster{bool, bool})
                n383 = Unbundle(w459) -> (w458:bool)  [unwired: 1 out]
                n384 = stacked-sequence {
                  tunnel: w458 -> [w462]
                  frame #0 {
                    n385 = case shown="False" w462 {
                      frame False {
                        n386 = local read "Completed 10"() -> (w463:bool)
                        n387 = case shown="True" w463 {
                          frame False {
                            n388 = property on="Completed 10" class="Bool (strict)"("Disabled"=u8 0) -> ()  [unwired: 2 in, 2 out]
                          }
                          frame True {
                            n389 = local write "Remind 10"(FALSE ("y")) -> ()
                            n390 = property on="Completed 10" class="Bool (strict)"("Disabled"=u8 1) -> ()  [unwired: 2 in, 2 out]
                          }
                        }
                      }
                      frame True {
                      }
                    }
                  }
                }
              }
              frame #10 {
                n391 = Index Array(array=w470, index=0) -> (element=w468:cluster{bool, bool})
                n392 = Unbundle(w468) -> (w467:bool)  [unwired: 1 out]
                n393 = stacked-sequence {
                  tunnel: w467 -> [w471]
                  frame #0 {
                    n394 = case shown="False" w471 {
                      frame False {
                        n395 = local read "Remind 1"() -> (w472:bool)
                        n396 = case shown="True" w472 {
                          frame False {
                            n397 = property on="Remind 1" class="Bool (strict)"("Disabled"=u8 0) -> ()  [unwired: 2 in, 2 out]
                          }
                          frame True {
                            n398 = local write "Completed 1"(FALSE ("y")) -> ()
                            n399 = property on="Remind 1" class="Bool (strict)"("Disabled"=u8 1) -> ()  [unwired: 2 in, 2 out]
                          }
                        }
                      }
                      frame True {
                      }
                    }
                  }
                }
              }
              frame #11 {
                n400 = Index Array(array=w479, index=1) -> (element=w477:cluster{bool, bool})
                n401 = Unbundle(w477) -> (w476:bool)  [unwired: 1 out]
                n402 = stacked-sequence {
                  tunnel: w476 -> [w480]
                  frame #0 {
                    n403 = case shown="False" w480 {
                      frame False {
                        n404 = local read "Remind 2"() -> (w481:bool)
                        n405 = case shown="True" w481 {
                          frame False {
                            n406 = property on="Remind 2" class="Bool (strict)"("Disabled"=u8 0) -> ()  [unwired: 2 in, 2 out]
                          }
                          frame True {
                            n407 = local write "Completed 2"(FALSE ("y")) -> ()
                            n408 = property on="Remind 2" class="Bool (strict)"("Disabled"=u8 1) -> ()  [unwired: 2 in, 2 out]
                          }
                        }
                      }
                      frame True {
                      }
                    }
                  }
                }
              }
              frame #12 {
                n409 = Index Array(array=w488, index=2) -> (element=w486:cluster{bool, bool})
                n410 = Unbundle(w486) -> (w485:bool)  [unwired: 1 out]
                n411 = stacked-sequence {
                  tunnel: w485 -> [w489]
                  frame #0 {
                    n412 = case shown="False" w489 {
                      frame False {
                        n413 = local read "Remind 3"() -> (w490:bool)
                        n414 = case shown="False" w490 {
                          frame False {
                            n415 = property on="Remind 3" class="Bool (strict)"("Disabled"=u8 0) -> ()  [unwired: 2 in, 2 out]
                          }
                          frame True {
                            n416 = local write "Completed 3"(FALSE ("y")) -> ()
                            n417 = property on="Remind 3" class="Bool (strict)"("Disabled"=u8 1) -> ()  [unwired: 2 in, 2 out]
                          }
                        }
                      }
                      frame True {
                      }
                    }
                  }
                }
              }
              frame #13 {
                n418 = Index Array(array=w497, index=3) -> (element=w495:cluster{bool, bool})
                n419 = Unbundle(w495) -> (w494:bool)  [unwired: 1 out]
                n420 = stacked-sequence {
                  tunnel: w494 -> [w498]
                  frame #0 {
                    n421 = case shown="False" w498 {
                      frame False {
                        n422 = local read "Remind 4"() -> (w499:bool)
                        n423 = case shown="False" w499 {
                          frame False {
                            n424 = property on="Remind 4" class="Bool (strict)"("Disabled"=u8 0) -> ()  [unwired: 2 in, 2 out]
                          }
                          frame True {
                            n425 = local write "Completed 4"(FALSE ("y")) -> ()
                            n426 = property on="Remind 4" class="Bool (strict)"("Disabled"=u8 1) -> ()  [unwired: 2 in, 2 out]
                          }
                        }
                      }
                      frame True {
                      }
                    }
                  }
                }
              }
              frame #14 {
                n427 = Index Array(array=w506, index=4) -> (element=w504:cluster{bool, bool})
                n428 = Unbundle(w504) -> (w503:bool)  [unwired: 1 out]
                n429 = stacked-sequence {
                  tunnel: w503 -> [w507]
                  frame #0 {
                    n430 = case shown="False" w507 {
                      frame False {
                        n431 = local read "Remind 5"() -> (w508:bool)
                        n432 = case shown="False" w508 {
                          frame False {
                            n433 = property on="Remind 5" class="Bool (strict)"("Disabled"=u8 0) -> ()  [unwired: 2 in, 2 out]
                          }
                          frame True {
                            n434 = local write "Completed 5"(FALSE ("y")) -> ()
                            n435 = property on="Remind 5" class="Bool (strict)"("Disabled"=u8 1) -> ()  [unwired: 2 in, 2 out]
                          }
                        }
                      }
                      frame True {
                      }
                    }
                  }
                }
              }
              frame #15 {
                n436 = Index Array(array=w515, index=5) -> (element=w513:cluster{bool, bool})
                n437 = Unbundle(w513) -> (w512:bool)  [unwired: 1 out]
                n438 = stacked-sequence {
                  tunnel: w512 -> [w516]
                  frame #0 {
                    n439 = case shown="False" w516 {
                      frame False {
                        n440 = local read "Remind 6"() -> (w517:bool)
                        n441 = case shown="False" w517 {
                          frame False {
                            n442 = property on="Remind 6" class="Bool (strict)"("Disabled"=u8 0) -> ()  [unwired: 2 in, 2 out]
                          }
                          frame True {
                            n443 = local write "Completed 6"(FALSE ("y")) -> ()
                            n444 = property on="Remind 6" class="Bool (strict)"("Disabled"=u8 1) -> ()  [unwired: 2 in, 2 out]
                          }
                        }
                      }
                      frame True {
                      }
                    }
                  }
                }
              }
              frame #16 {
                n445 = Index Array(array=w524, index=6) -> (element=w522:cluster{bool, bool})
                n446 = Unbundle(w522) -> (w521:bool)  [unwired: 1 out]
                n447 = stacked-sequence {
                  tunnel: w521 -> [w525]
                  frame #0 {
                    n448 = case shown="False" w525 {
                      frame False {
                        n449 = local read "Remind 7"() -> (w526:bool)
                        n450 = case shown="False" w526 {
                          frame False {
                            n451 = property on="Remind 7" class="Bool (strict)"("Disabled"=u8 0) -> ()  [unwired: 2 in, 2 out]
                          }
                          frame True {
                            n452 = local write "Completed 7"(FALSE ("y")) -> ()
                            n453 = property on="Remind 7" class="Bool (strict)"("Disabled"=u8 1) -> ()  [unwired: 2 in, 2 out]
                          }
                        }
                      }
                      frame True {
                      }
                    }
                  }
                }
              }
              frame #17 {
                n454 = Index Array(array=w533, index=7) -> (element=w531:cluster{bool, bool})
                n455 = Unbundle(w531) -> (w530:bool)  [unwired: 1 out]
                n456 = stacked-sequence {
                  tunnel: w530 -> [w534]
                  frame #0 {
                    n457 = case shown="False" w534 {
                      frame False {
                        n458 = local read "Remind 8"() -> (w535:bool)
                        n459 = case shown="False" w535 {
                          frame False {
                            n460 = property on="Remind 8" class="Bool (strict)"("Disabled"=u8 0) -> ()  [unwired: 2 in, 2 out]
                          }
                          frame True {
                            n461 = local write "Completed 8"(FALSE ("y")) -> ()
                            n462 = property on="Remind 8" class="Bool (strict)"("Disabled"=u8 1) -> ()  [unwired: 2 in, 2 out]
                          }
                        }
                      }
                      frame True {
                      }
                    }
                  }
                }
              }
              frame #18 {
                n463 = Index Array(array=w542, index=8) -> (element=w540:cluster{bool, bool})
                n464 = Unbundle(w540) -> (w539:bool)  [unwired: 1 out]
                n465 = stacked-sequence {
                  tunnel: w539 -> [w543]
                  frame #0 {
                    n466 = case shown="False" w543 {
                      frame False {
                        n467 = local read "Remind 9"() -> (w544:bool)
                        n468 = case shown="False" w544 {
                          frame False {
                            n469 = property on="Remind 9" class="Bool (strict)"("Disabled"=u8 0) -> ()  [unwired: 2 in, 2 out]
                          }
                          frame True {
                            n470 = local write "Completed 9"(FALSE ("y")) -> ()
                            n471 = property on="Remind 9" class="Bool (strict)"("Disabled"=u8 1) -> ()  [unwired: 2 in, 2 out]
                          }
                        }
                      }
                      frame True {
                      }
                    }
                  }
                }
              }
              frame #19 {
                n472 = Index Array(array=w551, index=9) -> (element=w549:cluster{bool, bool})
                n473 = Unbundle(w549) -> (w548:bool)  [unwired: 1 out]
                n474 = stacked-sequence {
                  tunnel: w548 -> [w552]
                  frame #0 {
                    n475 = case shown="False" w552 {
                      frame False {
                        n476 = local read "Remind 10"() -> (w553:bool)
                        n477 = case shown="False" w553 {
                          frame False {
                            n478 = property on="Remind 10" class="Bool (strict)"("Disabled"=u8 0) -> ()  [unwired: 2 in, 2 out]
                          }
                          frame True {
                            n479 = local write "Completed 10"(FALSE ("y")) -> ()
                            n480 = property on="Remind 10" class="Bool (strict)"("Disabled"=u8 1) -> ()  [unwired: 2 in, 2 out]
                          }
                        }
                      }
                      frame True {
                      }
                    }
                  }
                }
              }
              frame #20 {
                n481 = Bundle By Name(cluster=cluster{"Completed 1":bool, "Remind 1":bool} {"Completed 1"=FALSE, "Remind 1"=FALSE} ("input cluster"), "Completed 1"="Completed 1", "Remind 1"="Remind 1") -> (w557:cluster{"Completed 1":bool, "Remind 1":bool})
              }
              frame #21 {
                n482 = Bundle By Name(cluster=cluster{"Completed 2":bool, "Remind 2":bool} {"Completed 2"=FALSE, "Remind 2"=FALSE} ("input cluster"), "Completed 2"="Completed 2", "Remind 2"="Remind 2") -> (w563:cluster{"Completed 2":bool, "Remind 2":bool})
              }
              frame #22 {
                n483 = Bundle By Name(cluster=cluster{"Completed 3":bool, "Remind 3":bool} {"Completed 3"=FALSE, "Remind 3"=FALSE} ("input cluster"), "Completed 3"="Completed 3", "Remind 3"="Remind 3") -> (w565:cluster{"Completed 3":bool, "Remind 3":bool})
              }
              frame #23 {
                n484 = Bundle By Name(cluster=cluster{"Completed 4":bool, "Remind 4":bool} {"Completed 4"=FALSE, "Remind 4"=FALSE} ("input cluster"), "Completed 4"="Completed 4", "Remind 4"="Remind 4") -> (w569:cluster{"Completed 4":bool, "Remind 4":bool})
              }
              frame #24 {
                n485 = Bundle By Name(cluster=cluster{"Completed 5":bool, "Remind 5":bool} {"Completed 5"=FALSE, "Remind 5"=FALSE} ("input cluster"), "Completed 5"="Completed 5", "Remind 5"="Remind 5") -> (w573:cluster{"Completed 5":bool, "Remind 5":bool})
              }
              frame #25 {
                n486 = Bundle By Name(cluster=cluster{"Completed 6":bool, "Remind 6":bool} {"Completed 6"=FALSE, "Remind 6"=FALSE} ("input cluster"), "Completed 6"="Completed 6", "Remind 6"="Remind 6") -> (w577:cluster{"Completed 6":bool, "Remind 6":bool})
              }
              frame #26 {
                n487 = Bundle By Name(cluster=cluster{"Completed 7":bool, "Remind 7":bool} {"Completed 7"=FALSE, "Remind 7"=FALSE} ("input cluster"), "Completed 7"="Completed 7", "Remind 7"="Remind 7") -> (w581:cluster{"Completed 7":bool, "Remind 7":bool})
              }
              frame #27 {
                n488 = Bundle By Name(cluster=cluster{"Completed 8":bool, "Remind 8":bool} {"Completed 8"=FALSE, "Remind 8"=FALSE} ("input cluster"), "Completed 8"="Completed 8", "Remind 8"="Remind 8") -> (w585:cluster{"Completed 8":bool, "Remind 8":bool})
              }
              frame #28 {
                n489 = Bundle By Name(cluster=cluster{"Completed 9":bool, "Remind 9":bool} {"Completed 9"=FALSE, "Remind 9"=FALSE} ("input cluster"), "Completed 9"="Completed 9", "Remind 9"="Remind 9") -> (w589:cluster{"Completed 9":bool, "Remind 9":bool})
              }
              frame #29 {
                n490 = Bundle By Name(cluster=cluster{"Completed 10":bool, "Remind 10":bool} {"Completed 10"=FALSE, "Remind 10"=FALSE} ("input cluster"), "Completed 10"="Completed 10", "Remind 10"="Remind 10") -> (w593:cluster{"Completed 10":bool, "Remind 10":bool})
              }
            }
            n491 = Build Array(w365, w376, w375, w374, w373, w372, w371, w370, w369, w368) -> (w367:cluster{"Completed 10":bool, "Remind 10":bool}[])
          }
          frame #1 {
            n492 = for {
              tunnel: w600 -> [w604] mode=indexing
              tunnel: [w603] -> w597 mode=indexing
              tunnel: [w602] -> w599 mode=indexing
              tunnel: [w601] -> w598 mode=indexing
              i -> [w605]
              n493 = case shown="9" w605 {
                tunnel: w604 -> [_ w613 w618 w623 w628 w633 w638 w643 w648 w653 w658]
                tunnel: [TRUE w609 w614 w619 w624 w629 w634 w639 w644 w649 w654] -> w603
                tunnel: [FALSE w612 w617 w622 w627 w632 w637 w642 w647 w652 w657] -> w602
                tunnel: [TRUE w611 w616 w621 w626 w631 w636 w641 w646 w651 w656] -> w601
                frame -1, Default {
                }
                frame 0 {
                  n494 = Unbundle(w613) -> ("Completed 10"=w612:bool, "Remind 10"=w611:bool)
                  n495 = local write "Completed 1"(w612) -> ()
                  n496 = local write "Remind 1"(w611) -> ()
                  n497 = Or(x=w612, y=w611) -> (x .or. y?=w609:bool)
                  n498 = Not(x=w609) -> (.not. x?=w610:bool)
                  n499 = property on="Date 1" class="Str"("Blinking"=w610) -> ()  [unwired: 2 in, 2 out]
                }
                frame 1 {
                  n500 = Unbundle(w618) -> ("Completed 10"=w617:bool, "Remind 10"=w616:bool)
                  n501 = local write "Completed 2"(w617) -> ()
                  n502 = local write "Remind 2"(w616) -> ()
                  n503 = Or(x=w617, y=w616) -> (x .or. y?=w614:bool)
                  n504 = Not(x=w614) -> (.not. x?=w615:bool)
                  n505 = property on="Date 2" class="Str"("Blinking"=w615) -> ()  [unwired: 2 in, 2 out]
                }
                frame 2 {
                  n506 = Unbundle(w623) -> ("Completed 10"=w622:bool, "Remind 10"=w621:bool)
                  n507 = local write "Completed 3"(w622) -> ()
                  n508 = local write "Remind 3"(w621) -> ()
                  n509 = Or(x=w622, y=w621) -> (x .or. y?=w619:bool)
                  n510 = Not(x=w619) -> (.not. x?=w620:bool)
                  n511 = property on="Date 3" class="Str"("Blinking"=w620) -> ()  [unwired: 2 in, 2 out]
                }
                frame 3 {
                  n512 = Unbundle(w628) -> ("Completed 10"=w627:bool, "Remind 10"=w626:bool)
                  n513 = local write "Completed 4"(w627) -> ()
                  n514 = local write "Remind 4"(w626) -> ()
                  n515 = Or(x=w627, y=w626) -> (x .or. y?=w624:bool)
                  n516 = Not(x=w624) -> (.not. x?=w625:bool)
                  n517 = property on="Date 4" class="Str"("Blinking"=w625) -> ()  [unwired: 2 in, 2 out]
                }
                frame 4 {
                  n518 = Unbundle(w633) -> ("Completed 10"=w632:bool, "Remind 10"=w631:bool)
                  n519 = local write "Completed 5"(w632) -> ()
                  n520 = local write "Remind 5"(w631) -> ()
                  n521 = Or(x=w632, y=w631) -> (x .or. y?=w629:bool)
                  n522 = Not(x=w629) -> (.not. x?=w630:bool)
                  n523 = property on="Date 5" class="Str"("Blinking"=w630) -> ()  [unwired: 2 in, 2 out]
                }
                frame 5 {
                  n524 = Unbundle(w638) -> ("Completed 10"=w637:bool, "Remind 10"=w636:bool)
                  n525 = local write "Completed 6"(w637) -> ()
                  n526 = local write "Remind 6"(w636) -> ()
                  n527 = Or(x=w637, y=w636) -> (x .or. y?=w634:bool)
                  n528 = Not(x=w634) -> (.not. x?=w635:bool)
                  n529 = property on="Date 6" class="Str"("Blinking"=w635) -> ()  [unwired: 2 in, 2 out]
                }
                frame 6 {
                  n530 = Unbundle(w643) -> ("Completed 10"=w642:bool, "Remind 10"=w641:bool)
                  n531 = local write "Completed 7"(w642) -> ()
                  n532 = local write "Remind 7"(w641) -> ()
                  n533 = Or(x=w642, y=w641) -> (x .or. y?=w639:bool)
                  n534 = Not(x=w639) -> (.not. x?=w640:bool)
                  n535 = property on="Date 7" class="Str"("Blinking"=w640) -> ()  [unwired: 2 in, 2 out]
                }
                frame 7 {
                  n536 = Unbundle(w648) -> ("Completed 10"=w647:bool, "Remind 10"=w646:bool)
                  n537 = local write "Completed 8"(w647) -> ()
                  n538 = local write "Remind 8"(w646) -> ()
                  n539 = Or(x=w647, y=w646) -> (x .or. y?=w644:bool)
                  n540 = Not(x=w644) -> (.not. x?=w645:bool)
                  n541 = property on="Date 8" class="Str"("Blinking"=w645) -> ()  [unwired: 2 in, 2 out]
                }
                frame 8 {
                  n542 = Unbundle(w653) -> ("Completed 10"=w652:bool, "Remind 10"=w651:bool)
                  n543 = local write "Completed 9"(w652) -> ()
                  n544 = local write "Remind 9"(w651) -> ()
                  n545 = Or(x=w652, y=w651) -> (x .or. y?=w649:bool)
                  n546 = Not(x=w649) -> (.not. x?=w650:bool)
                  n547 = property on="Date 9" class="Str"("Blinking"=w650) -> ()  [unwired: 2 in, 2 out]
                }
                frame 9 {
                  n548 = Unbundle(w658) -> ("Completed 10"=w657:bool, "Remind 10"=w656:bool)
                  n549 = local write "Completed 10"(w657) -> ()
                  n550 = local write "Remind 10"(w656) -> ()
                  n551 = Or(x=w657, y=w656) -> (x .or. y?=w654:bool)
                  n552 = Not(x=w654) -> (.not. x?=w655:bool)
                  n553 = property on="Date 10" class="Str"("Blinking"=w655) -> ()  [unwired: 2 in, 2 out]
                }
              }
            }
          }
          frame #2 {
            n554 = Search 1D Array(1D array=w659, element=FALSE) -> (index of element=w660:i32)  [unwired: 1 out]
            n555 = case shown="-1" w660 {
              frame 0, Default {
              }
              frame -1 {
                n556 = local read "No Alarms"() -> (w662:bool)
                n557 = case shown="True" w662 {
                  frame False {
                  }
                  frame True {
                    n558 = local write "Save"(TRUE ("element")) -> ()
                  }
                }
              }
            }
          }
          frame #3 {
            n559 = Wait (ms)(milliseconds to wait=u32 100) -> ()  [unwired: 1 out]
          }
          frame #4 {
            n560 = local read "Save"() -> (w668:bool)
            n561 = Search 1D Array(1D array=w670, element=FALSE) -> (index of element=w671:i32)  [unwired: 1 out]
            n562 = case shown="0, Default" w671 {
              tunnel: [w675 w676] -> w665
              tunnel: w668 -> [w675 w677]
              frame -1 {
              }
              frame 0, Default {
                w676 = FALSE ("Save")
                n563 = call "Display Message to User2"("Enable"=w677) -> ()  [unwired: 2 in, 9 out]
                n564 = local write "Save"(w676) -> ()
              }
            }
            n565 = local read "Edit File"() -> (w667:bool)
            n566 = case shown="False" w667 {
              tunnel: [w673 TRUE] -> w666
              tunnel: w665 -> [w673 _]
              frame False {
              }
              frame True {
              }
            }
            n567 = local write "No Alarms"(FALSE) -> ()
          }
        }
      }
    }
    frame #7 {
      n568 = case shown="False" w678 {
        tunnel: w683 -> [w688 _]
        tunnel: w682 -> [w687 _]
        tunnel: w681 -> [w686 _]
        tunnel: w680 -> [w685 _]
        tunnel: w679 -> [w684 _]
        frame False {
          # "New Sorted Data"
          # "Write to Key Values"
          # "Key Values"
          # "New data"
          # "Key Name"
          # "Temp Key Value"
          # "Saving values"
          n569 = stacked-sequence {
            seq-local: [_ w696 _ _ _ _ _ _] -> [_ _ w714 _ _ _ _ _]
            seq-local: [w689 _ _ _ _ _ _ _] -> [_ _ _ _ _ _ w746 _]
            seq-local: [w690 _ _ _ _ _ _ _] -> [_ _ _ _ w730 w742 _ _]
            seq-local: [_ _ w711 _ _ _ _ _] -> [_ _ _ w721 _ _ _ _]
            seq-local: [_ _ _ _ _ w741 _ _] -> [_ _ _ _ _ _ w747 _]
            seq-local: [_ _ _ _ w728 _ _ _] -> [_ _ _ _ _ w740 _ _]
            seq-local: [_ _ _ w720 _ _ _ _] -> [_ _ _ _ w727 _ _ _]
            tunnel: w688 -> [_ w700 _ _ _ _ _ _]
            tunnel: w687 -> [_ w699 _ w723 _ _ _ _]
            tunnel: w686 -> [_ w698 _ _ _ _ _ _]
            tunnel: w685 -> [_ _ w713 _ _ _ _ _]
            tunnel: w684 -> [_ _ w712 _ _ _ _ _]
            frame #0 {
              n570 = Initialize Array "Initialize Array"("", 1 ("dimension size"), 10 ("dimension size")) -> (w691:string[][])
              n571 = call "MC - Fill Default Values.vi"("Key Value In"=w691, "Key Name In"=w691, "Array of Bad Data"=i32[] [0, 1, 2, 3, 4, 5, 6, 7, 8, 9]) -> ("Key Value Out"=w690:string[][], "Key Name Out"=w689:string[][])
            }
            frame #1 {
              # "Add new dates if needed"
              n572 = Array Size(array=w699) -> (size(s)=w697:i32)
              n573 = for {
                N: w697 -> [_]
                tunnel: w700 -> [w704] mode=indexing
                shift-right: [w702] -> w696
                shift-left: w698 -> [w703]
                tunnel: w699 -> [w701] mode=indexing
                n574 = case shown="True" w704 {
                  tunnel: w703 -> [w705 w710]
                  tunnel: w701 -> [_ w709]
                  tunnel: [w705 w706] -> w702
                  frame False {
                  }
                  frame True {
                    n575 = Format Date/Time String(time format string (%c)="%m/%d/%Y") -> (date/time string=w707:string)  [unwired: 2 out]
                    n576 = Replace Array Subset(array=w710, new element=w707, index=w709) -> (w706:string[])
                  }
                }
              }
            }
            frame #2 {
              # "Put data in form for ballistic.ini file"
              # "date"
              # "message"
              # "interval"
              n577 = for {
                tunnel: w714 -> [w719] mode=indexing
                tunnel: w713 -> [w717] mode=indexing
                tunnel: w712 -> [w716] mode=indexing
                tunnel: [w715] -> w711 mode=indexing
                w718 = "&"
                n578 = Concatenate Strings(w719, w718, w717, w718, w716) -> (w715:string)
              }
            }
            frame #3 {
              # "Rearrange reminders by date"
              n579 = Array Size(array=w723) -> (size(s)=w722:i32)
              n580 = for {
                N: w722 -> [_]
                tunnel: w723 -> [w726] mode=indexing
                tunnel: w721 -> [w725]
                tunnel: [w724] -> w720 mode=indexing
                n581 = Index Array(array=w725, index=w726) -> (element=w724:string)
              }
            }
            frame #4 {
              # "Insert into Temp Key Value array"
              n582 = Array Size(array=w727) -> (size(s)=w729:i32)
              n583 = case shown="1.." w729 {
                tunnel: w730 -> [w732 w739]
                tunnel: w727 -> [_ w735]
                tunnel: [w731 w734] -> w728
                frame ..0 {
                  n584 = Index Array(array=w732, index (row)=0) -> (element=w731:string[])  [unwired: 1 in]
                }
                frame 1.. {
                  n585 = Index Array(array=w739, index (row)=0) -> (element=w737:string[])  [unwired: 1 in]
                  n586 = Replace Array Subset(array=w737, new element=w735, index=0) -> (w734:string[])
                }
              }
            }
            frame #5 {
              # "Make Key Value array"
              n587 = Replace Array Subset(array=w742, new element=w740, index (row)=0) -> (w741:string[][])  [unwired: 1 in]
            }
            frame #6 {
              # "write to ballistic.ini"
              n588 = local read "INI File Name"() -> (w744:string)
              n589 = call "MC - Create INI.vi"("INI File Name"=w744, "Fill Data"=TRUE, "Save File"=TRUE, "Key Value"=w747, "Key Name"=w746) -> ()  [unwired: 5 out]
            }
            frame #7 {
              n590 = flat-sequence {
                frame #0 {
                  n591 = local read "Edit File"() -> (w749:bool)
                  n592 = case shown="True" w749 {
                    frame False {
                    }
                    frame True {
                      # "edit ballistic.ini"
                      n593 = local read "INI File Name"() -> (w750:string)
                      n594 = call "MC - Create INI.vi"("INI File Name"=w750, "Save File"=FALSE) -> ()  [unwired: 3 in, 5 out]
                    }
                  }
                }
                frame #1 {
                  w752 = FALSE ("Save")
                  n595 = local write "No Alarms"(FALSE ("No Alarms")) -> ()
                  n596 = local write "Edit File"(w752) -> ()
                  n597 = local write "Save"(w752) -> ()
                }
              }
            }
          }
        }
        frame True {
        }
      }
    }
  }
  n598 = flat-sequence {
    tunnel: ["Section Name"] -> _
    tunnel: ["Date"] -> _
    tunnel: ["Edit File"] -> _
    tunnel: ["Key Name"] -> _
    tunnel: ["Interval in Days"] -> _
    tunnel: ["Save"] -> _
    tunnel: ["Key Value"] -> _
    tunnel: ["Message"] -> _
    tunnel: ["No Alarms"] -> _
    frame #0 {
    }
  }
  n599 = property on="Edit File" class="Bool (strict)"("Visible"=FALSE) -> ()  [unwired: 2 in, 2 out]
